vi "warehouse temperature control.vi"() -> ()   [LabVIEW 2020]
uses:
  <vilib>/MakerHub/LINX/Public/Peripherals/Analog/Analog Read 1 Chan.vi
  <vilib>/MakerHub/LINX/Public/Peripherals/Analog/Analog Read N Chans.vi
  <vilib>/MakerHub/LINX/Private/Local IO/LinxAnalogRead.vi
  <vilib>/MakerHub/LINX/Public/Utilities/Check Channel.vi
  <vilib>/MakerHub/LINX/Public/Utilities/Open Serial.vi
  <vilib>/MakerHub/LINX/Private/Utilties/Generate Error.vi
  <vilib>/smtpClient/Set Message Text.vi
  <vilib>/MakerHub/LINX/LMH-LINX.lvlib
  <vilib>/smtpClient/LabVIEWSMTPClient.lvlib
panel:
  in  "Sistem şifre":string
  in  "Sistem mail":string
  in  "Kanal":u8=2
  in  "Baud Rate Override":u32=9600
  in  "Seri port":refnum<visa-resource-name>="COM3"
  out "Alarm":string
  out "Sistem uyarısı":string
  out "Sıcaklık":dbl
  out "?":bool
  out "?":bool
  out "?":bool
  out "Soğutucular":string
  out "Sıcaklık":dbl(graph)
  # "Tehlike Durumu"
  # "URHAN MÜHENDİSLİK ve \nDANIŞMANLIK HİZMETLERİ"
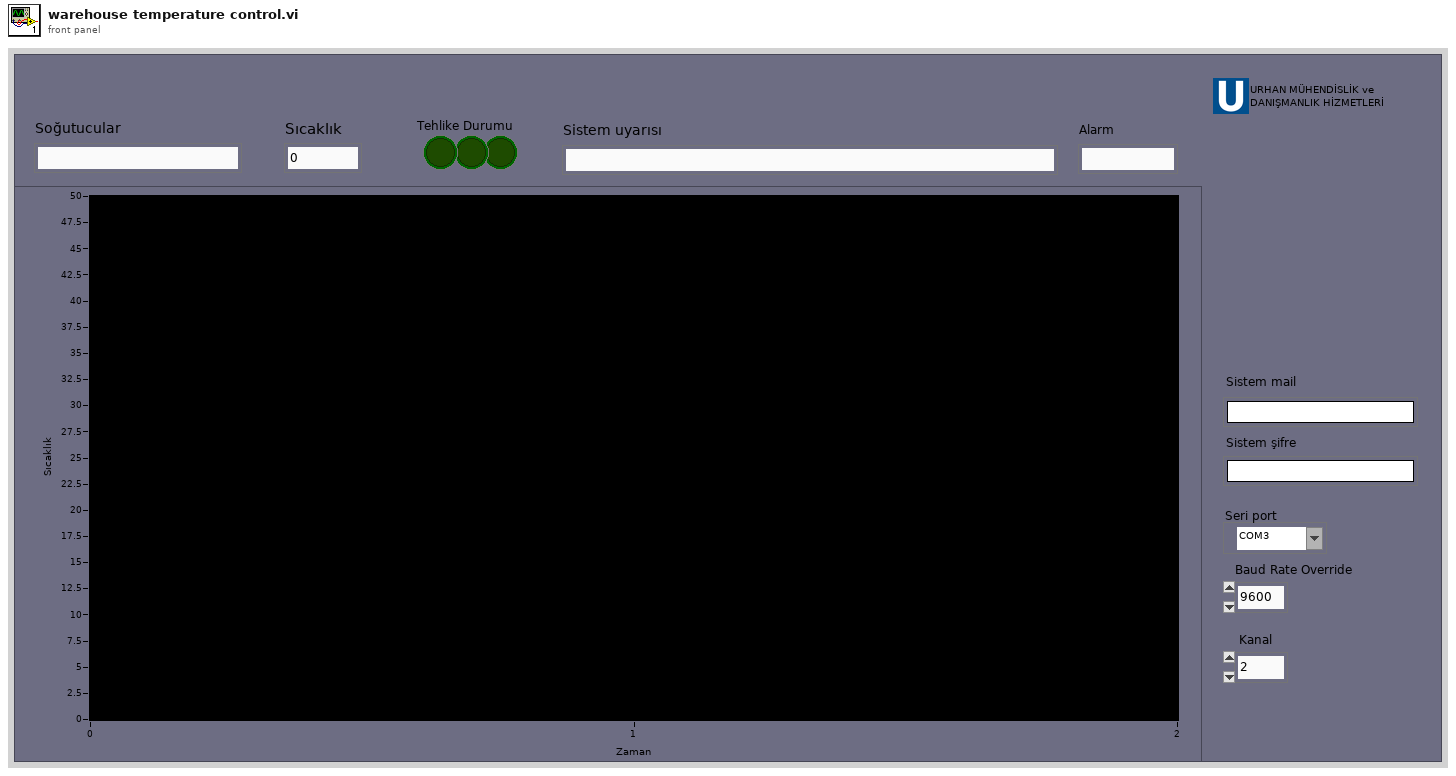
[diagram p1: front panel]
types:
  T1 = typedef "LMH-LINX.lvlib/LINX Ref.ctl" = cluster{"IO":T2, "Interface":T3, "LINX Device Config":T4}
  T2 = typedef "LMH-LINX.lvlib/Platform.ctl" = enum16{"Remote", "Local"}
  T3 = typedef "LMH-LINX.lvlib/Interface.ctl" = enum16{"Serial", "TCP"}
  T4 = typedef "LMH-LINX.lvlib/Device.lvlib/LINX Device Config.ctl" = cluster{"Interface":T3, "COM Port":refnum<visa-resource-name>, "TCP Configuration":T5, "Device Family":u8, "Device ID":u8, "Device Name":string, "TCP Ref":refnum<k5>, "Channels":T6}
  T5 = typedef "LMH-LINX.lvlib/Device.lvlib/TCP Config.ctl" = cluster{"IP Address":string, "Port":u16}
  T6 = typedef "LMH-LINX.lvlib/Channels.ctl" = cluster{"DI":u8[], "DO":u8[], "AI":u8[], "AO":u8[], "PWM":u8[], "QE":u8[], "UART":u8[], "I2C 2":u8[], "SPI":u8[], "CAN":u8[], "Servo":u8[], "AI Ref (V)":dbl, "AI Resolution (Bits)":u8, "AO Ref (V)":dbl, "AO Resolution (Bits)":u8}
  T7 = typedef "LabVIEWSMTPClient.lvlib/SmtpClientHandle.ctl" = refnum<k1>
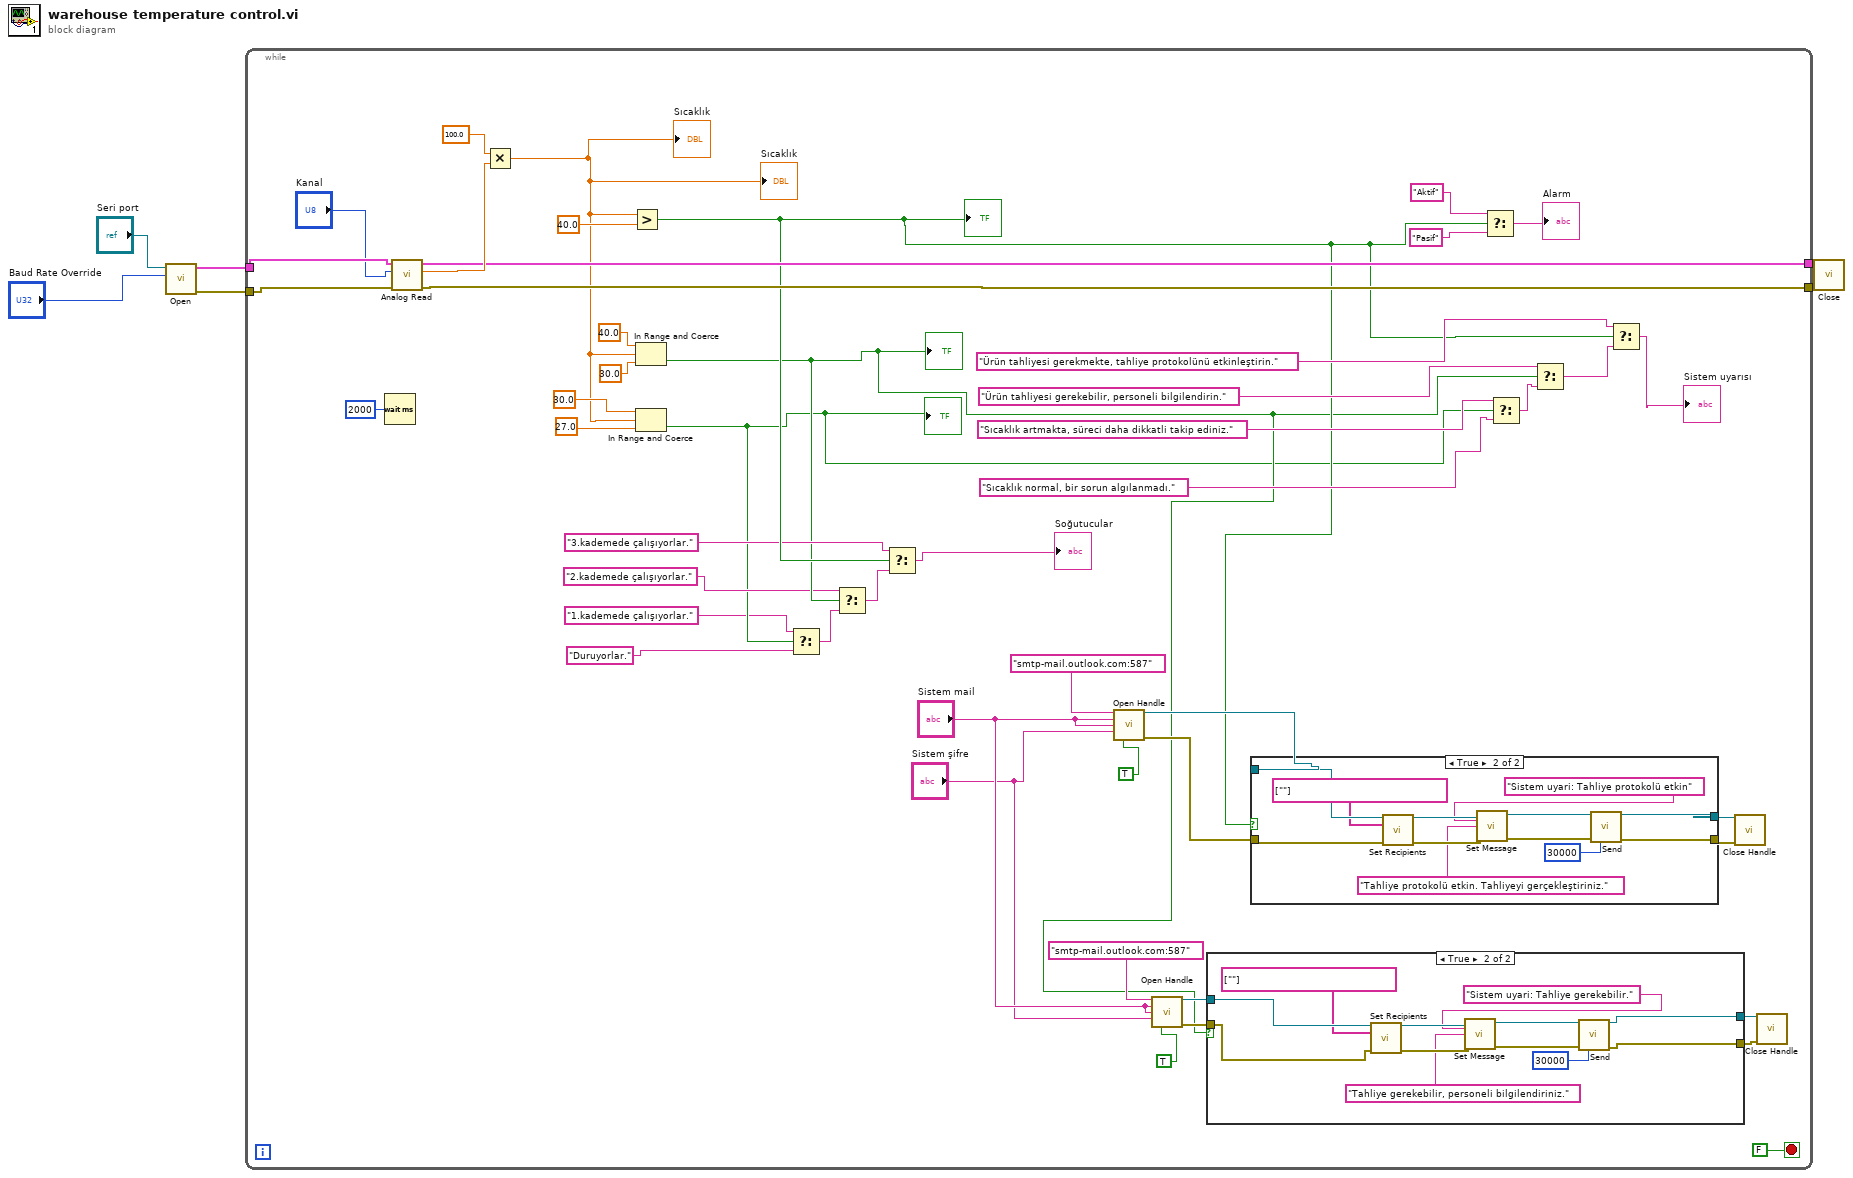
[diagram p0: block diagram]
diagram:
  n1 = call-poly <vilib>:"Open.vi"("Baud Rate Override"="Baud Rate Override", "Serial Port"="Seri port") -> ("Error Out"=w5:errorcluster, "LINX Resource"=w6:T1)  [unwired: 7 in, 1 out]
  n2 = while {
    tunnel: w6 -> [w52]
    tunnel: w5 -> [w51]
    tunnel: [w47] -> w2
    tunnel: [w46] -> w1
    stop <- FALSE stop-if-true
    n3 = Wait (ms)(milliseconds to wait=u32 2000) -> ()  [unwired: 1 out]
    n4 = call-poly <vilib>:"Analog Read.vi"("Error In"=w51, "Analog Channel"="Kanal", "LINX Resource"=w52) -> ("Error Out"=w46:errorcluster, "Voltage"=w55:dbl, "LINX Resource"=w47:T1)  [unwired: 5 in, 1 out]
    n5 = Multiply(x=100.0, y=w55) -> (x*y=w43:dbl)
    "Sıcaklık" <- w43
    "Sıcaklık" <- w43
    n6 = Greater?(x=w43, y=40.0) -> (0:w16:bool)
    "?" <- w16
    n7 = In Range and Coerce(upper limit=40.0, x=w43, lower limit=30.0) -> (In Range?=w13:bool)  [unwired: 1 out]
    "?" <- w13
    n8 = In Range and Coerce(upper limit=30.0, x=w43, lower limit=27.0 ("x")) -> (In Range?=w9:bool)  [unwired: 1 out]
    "?" <- w9
    n9 = Select(t="1.kademede çalışıyorlar.", s=w9, f="Duruyorlar.") -> (s? t:f=w10:string)
    n10 = Select(t="2.kademede çalışıyorlar.", s=w13, f=w10) -> (s? t:f=w12:string)
    n11 = Select(t="3.kademede çalışıyorlar.", s=w16, f=w12) -> (s? t:f=→"Soğutucular":string)
    n12 = call <vilib>:"Open Handle.vi"("server address"="smtp-mail.outlook.com:587", "from"="Sistem mail", "username"="Sistem mail", "password"="Sistem şifre", "use TLS (false)"=TRUE) -> ("handle out"=w28:T7, "error out"=w25:errorcluster)  [unwired: 9 in]
    n13 = call <vilib>:"Open Handle.vi"("server address"="smtp-mail.outlook.com:587", "from"="Sistem mail", "username"="Sistem mail", "password"="Sistem şifre", "use TLS (false)"=TRUE) -> ("handle out"=w18:T7, "error out"=w17:errorcluster)  [unwired: 9 in]
    n14 = case shown="True" w13 {
      tunnel: [w57 w59] -> w20
      tunnel: [w56 w60] -> w19
      tunnel: w18 -> [w57 w62]
      tunnel: w17 -> [w56 w61]
      frame False {
      }
      frame True {
        n15 = call <vilib>:"Set Recipients.vi"("handle in"=w62, "to"=string[] [""], "error in (no error)"=w61) -> ("handle out"=w69:T7, "error out"=w67:errorcluster)  [unwired: 11 in]
        n16 = call-poly <vilib>:"Set Message.vi"("handle in"=w69, "subject"="Sistem uyari: Tahliye gerekebilir.", "plain text message"="Tahliye gerekebilir, personeli bilgilendiriniz.", "error in (no error)"=w67) -> ("handle out"=w68:T7, "error out"=w66:errorcluster)  [unwired: 10 in]
        n17 = call <vilib>:"Send.vi"("handle in"=w68, "error in (no error)"=w66, "timeout in ms (10000)"=30000) -> ("handle out"=w59:T7, "error out"=w60:errorcluster)  [unwired: 10 in, 1 out]
      }
    }
    n18 = case shown="True" w16 {
      tunnel: w28 -> [w71 w81]
      tunnel: [w71 w80] -> w27
      tunnel: [w70 w77] -> w26
      tunnel: w25 -> [w70 w73]
      frame False {
      }
      frame True {
        n19 = call <vilib>:"Set Recipients.vi"("handle in"=w81, "to"=string[] [""], "error in (no error)"=w73) -> ("handle out"=w83:T7, "error out"=w79:errorcluster)  [unwired: 11 in]
        n20 = call-poly <vilib>:"Set Message.vi"("handle in"=w83, "subject"="Sistem uyari: Tahliye protokolü etkin", "plain text message"="Tahliye protokolü etkin. Tahliyeyi gerçekleştiriniz.", "error in (no error)"=w79) -> ("handle out"=w82:T7, "error out"=w78:errorcluster)  [unwired: 10 in]
        n21 = call <vilib>:"Send.vi"("handle in"=w82, "error in (no error)"=w78, "timeout in ms (10000)"=30000) -> ("handle out"=w80:T7, "error out"=w77:errorcluster)  [unwired: 10 in, 1 out]
      }
    }
    n22 = Select(t="Aktif", s=w16, f="Pasif") -> (s? t:f=→"Alarm":string)
    n23 = Select(t="Sıcaklık artmakta, süreci daha dikkatli takip ediniz.", s=w9, f="Sıcaklık normal, bir sorun algılanmadı.") -> (s? t:f=w38:string)
    n24 = Select(t="Ürün tahliyesi gerekebilir, personeli bilgilendirin.", s=w13, f=w38) -> (s? t:f=w36:string)
    n25 = Select(t="Ürün tahliyesi gerekmekte, tahliye protokolünü etkinleştirin.", s=w16, f=w36) -> (s? t:f=→"Sistem uyarısı":string)
    n26 = call <vilib>:"Close Handle.vi"("handle in"=w27, "error in (no error)"=w26) -> ()  [unwired: 12 in, 2 out]
    n27 = call <vilib>:"Close Handle.vi"("handle in"=w20, "error in (no error)"=w19) -> ()  [unwired: 12 in, 2 out]
  }
  n28 = call <vilib>:"Close.vi"("Error In"=w1, "LINX Resource"=w2) -> ()  [unwired: 9 in, 1 out]
